vi "FGV_temp.vi"(6 "R/W":enum16{"Read", "Write"}(ring)=enum."Write", 8 "error":errorcluster, 10 "value":dbl, 11 "Temperature in":cluster{cluster{"Xi":dbl, "Yi":dbl}[]}[](graph) caption="Temperature") -> (0 "error  out":errorcluster, 2 "Value out":dbl, 3 "Temp out":cluster{cluster{"Xi":dbl, "Yi":dbl}[]}[](array[cluster]))   [LabVIEW 2022 SP3]
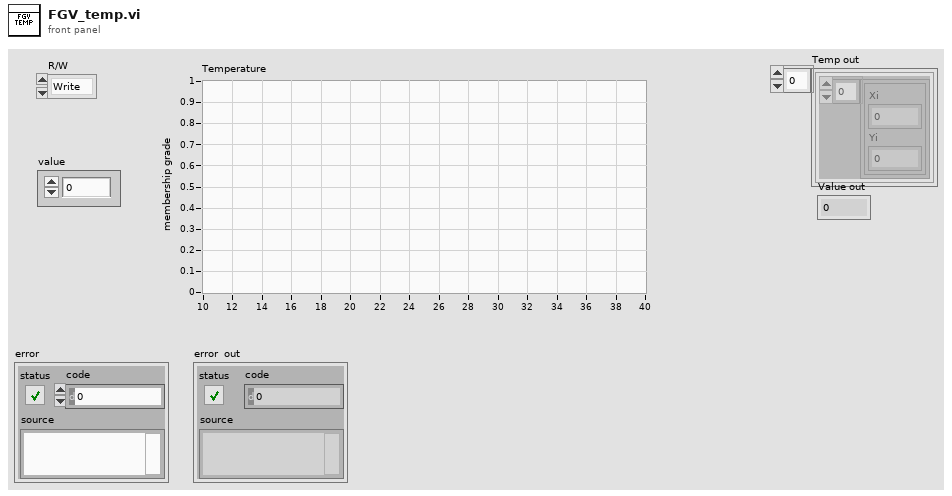
[diagram p1: front panel]
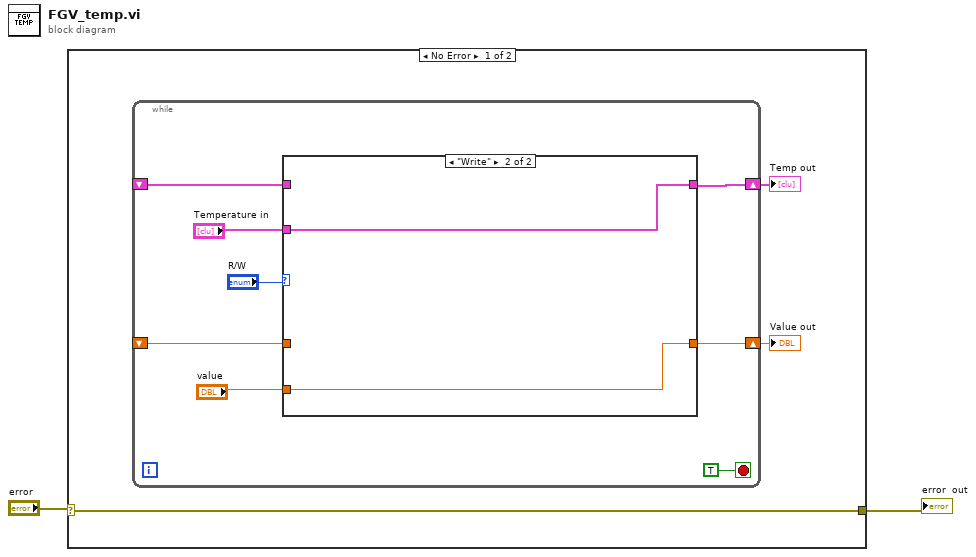
[diagram p0: block diagram]
diagram:
  n1 = case shown="No Error" "error" {
    selector: "error" -> [w5 w18]
    tunnel: [w5 w18] -> w1
    frame No Error {
      n2 = while {
        shift-right: [w11] -> w4
        shift-left: _ -> [w9]
        shift-right: [w8] -> w3
        shift-left: _ -> [w6]
        stop <- TRUE stop-if-true
        n3 = case shown="\"Write\"" "R/W" {
          tunnel: [w15 w17] -> w11
          tunnel: "Temperature in" -> [_ w17]
          tunnel: w9 -> [w15 _]
          tunnel: [w14 w16] -> w8
          tunnel: "value" -> [_ w16]
          tunnel: w6 -> [w14 _]
          frame "Read", Default {
          }
          frame "Write" {
          }
        }
      }
      "Temp out" <- w4
      "Value out" <- w3
    }
    frame Error {
    }
  }
  "error  out" <- w1
